vi "Flatten Cluster To CfgTable.vi"(8 "error in (no error)":errorcluster, 11 "Cluster Configuration Typedef":variant) -> (0 "error out":errorcluster, 3 "CfgTable Row":string[](array[string]))   [LabVIEW 2017, in "ClusterCfgTable.lvlib"]
uses:
  ClusterCfgTable.lvlib
panel:
  in  "ConfigStrings Typedef":string[](array[string])
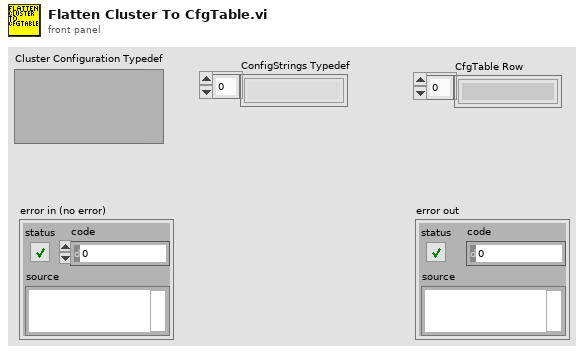
[diagram p1: front panel]
types:
  T1 = typedef "Type Descriptor Enumeration__ogtk.ctl" = enum8{"<Null>", "I8", "I16", "I32", "I64", "U8", "U16", "U32", "U64", "SGL", "DBL", "EXT", "CSG", "CDB", "CXT", "0x0F", "0x10", "0x11", "0x12", "0x13", "0x14", "Enum U8", "Enum U16", "Enum U32", "Enum U64", "SGL PQ", "DBL PQ", "EXT PQ", "CSG PQ", "CDB PQ", "CXT PQ", "0x1F", "0x20", "Boolean", "0x22", "0x23", "0x24", "0x25", "0x26", "0x27", "0x28", "0x29", "0x2A", "0x2B", "0x2C", "0x2D", "0x2E", "0x2F", "String", "0x31", "Path", "Pict", "0x34", "0x35", "0x36", "DAQ", "0x38", "0x39", "0x3A", "0x3B", "0x3C", "0x3D", "0x3E", "0x3F", "Array", "0x41", "0x42", "0x43", "0x44", "0x45", "0x46", "0x47", "0x48", "0x49", "0x4A", "0x4B", "0x4C", "0x4D", "0x4E", "0x4F", "Cluster", "0x51", "0x52", "Variant", "Waveform", "0x55", "0x56", "0x57", "0x58", "0x59", "0x5A", "0x5B", "0x5C", "0x5D", "0x5E", "0x5F", "0x60", "0x61", "0x62", "0x63", "0x64", "0x65", "0x66", "0x67", "0x68", "0x69", "0x6A", "0x6B", "0x6C", "0x6D", "0x6E", "0x6F", "Refnum"}
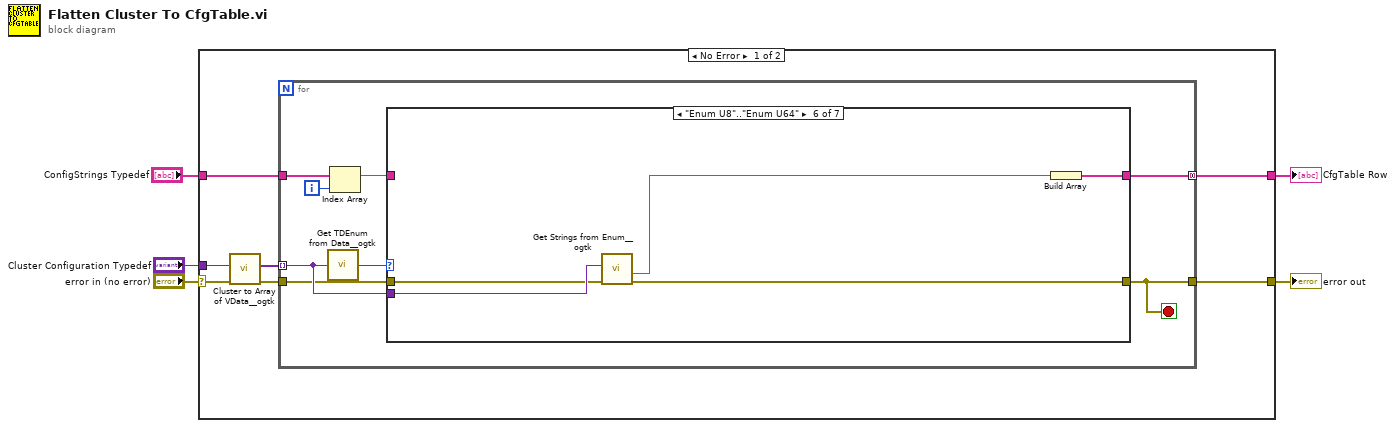
[diagram p0: block diagram]
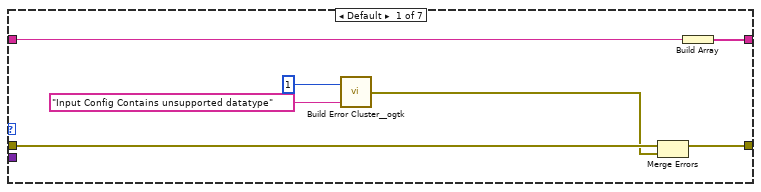
[diagram p2: hidden frame]
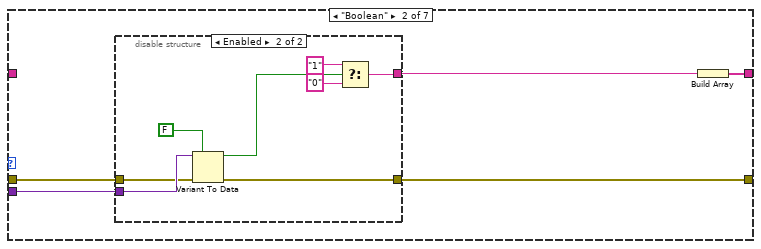
[diagram p3: hidden frame]
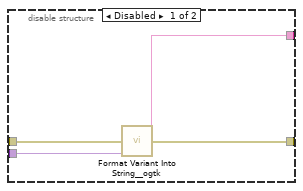
[diagram p4: hidden frame]
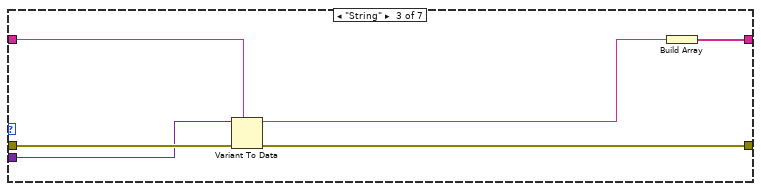
[diagram p5: hidden frame]
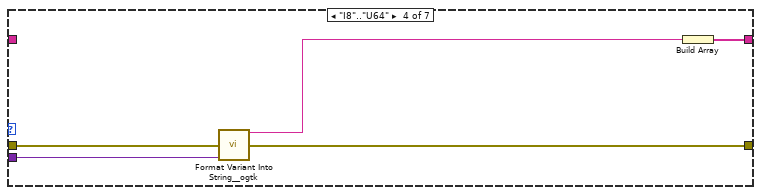
[diagram p6: hidden frame]
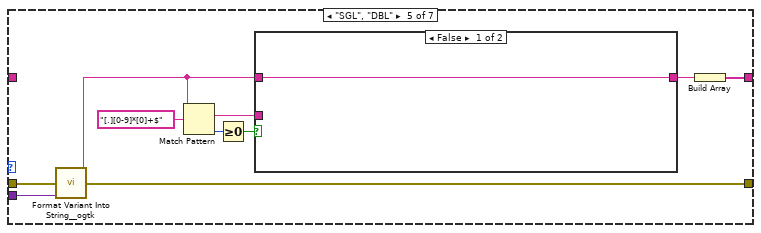
[diagram p7: hidden frame]
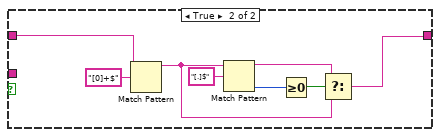
[diagram p8: hidden frame]
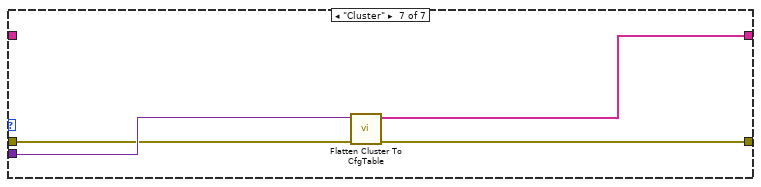
[diagram p9: hidden frame]
diagram:
  n1 = case shown="No Error" "error in (no error)" {
    selector: "error in (no error)" -> [w10 w85]
    tunnel: [w12 w85] -> w5
    tunnel: "Cluster Configuration Typedef" -> [w8 _]
    tunnel: [w7 w84] -> w2
    tunnel: "ConfigStrings Typedef" -> [w6 w84]
    frame No Error {
      n2 = call <userlib>:"Cluster to Array of VData__ogtk.vi"("error in (no error)"=w10, "Cluster"=w8) -> ("error out"=w11:errorcluster, "Array of VData"=w9:variant[])  [unwired: 8 in]
      n3 = for {
        tunnel: w9 -> [w19] mode=indexing
        tunnel: w11 -> [w18]
        tunnel: [w17] -> w12
        tunnel: [w16] -> w7 mode=concatenating
        tunnel: w6 -> [w15]
        i -> [w13]
        stop <- w17 stop-if-true
        n4 = call <userlib>:"Get TDEnum from Data__ogtk.vi"("Data"=w19) -> ("Type Descriptor Enumeration"=w20:T1)  [unwired: 4 in]
        n5 = Index Array(array=w15, index=w13) -> (element=w14:string)
        n6 = case shown="\"Enum U8\"..\"Enum U64\"" w20 {
          tunnel: w19 -> [_ w31 w48 w53 w59 w79 w83]
          tunnel: w18 -> [w27 w32 w50 w55 w60 w78 w81]
          tunnel: [w26 w29 w49 w54 w58 w76 w80] -> w17
          tunnel: [w21 w28 w45 w51 w56 w75 w82] -> w16
          tunnel: w14 -> [w22 _ w47 _ _ _ _]
          frame Default {
            n7 = call <userlib>:"Build Error Cluster__ogtk.vi"("String to Prepend to source (\"\")"="Input Config Contains unsupported datatype" ("String to Prepend to source (\"\")"), "code"=1) -> ("error out"=w25:errorcluster)
            n8 = Merge Errors(w27, w25) -> (w26:errorcluster)
            n9 = Build Array(w22) -> (w21:string[])
          }
          frame "Boolean" {
            n10 = disable-structure shown="Enabled" {
              disable-tunnel: w31 -> [w36 w44]
              disable-tunnel: w32 -> [w35 w43]
              disable-tunnel: [w34 w42] -> w29
              disable-tunnel: [w33 w39] -> w30
              frame Disabled {
                n11 = call <userlib>:"Format Variant Into String__ogtk.vi"("error in (no error)"=w35, "Variant"=w36) -> ("Output String"=w33:string, "error out"=w34:errorcluster)  [unwired: 12 in]
              }
              frame Enabled {
                n12 = Variant To Data(error in=w43, type=FALSE, Variant=w44) -> (data=w40:bool, error out=w42:errorcluster)
                n13 = Select(t="1", s=w40, f="0") -> (s? t:f=w39:string)
              }
            }
            n14 = Build Array(w30) -> (w28:string[])
          }
          frame "String" {
            n15 = Variant To Data(error in=w50, type=w47, Variant=w48) -> (data=w46:string, error out=w49:errorcluster)
            n16 = Build Array(w46) -> (w45:string[])
          }
          frame "I8".."U64" {
            n17 = call <userlib>:"Format Variant Into String__ogtk.vi"("error in (no error)"=w55, "Variant"=w53) -> ("Output String"=w52:string, "error out"=w54:errorcluster)  [unwired: 12 in]
            n18 = Build Array(w52) -> (w51:string[])
          }
          frame "SGL", "DBL" {
            n19 = call <userlib>:"Format Variant Into String__ogtk.vi"("error in (no error)"=w60, "Variant"=w59) -> ("Output String"=w62:string, "error out"=w58:errorcluster)  [unwired: 12 in]
            n20 = Match Pattern(string=w62, regular expression="[.][0-9]*[0]+$") -> (match substring=w61:string, offset past match=w64:i32)  [unwired: 1 in, 2 out]
            n21 = Greater Or Equal To 0?(x=w64) -> (x >= 0?=w63:bool)
            n22 = case shown="False" w63 {
              tunnel: [w66 w74] -> w57
              tunnel: w62 -> [w66 w72]
              tunnel: w61 -> [_ _]
              frame False {
              }
              frame True {
                n23 = Match Pattern(string=w72, regular expression="[0]+$") -> (before substring=w71:string)  [unwired: 1 in, 3 out]
                n24 = Match Pattern(string=w71, regular expression="[.]$") -> (before substring=w67:string, offset past match=w69:i32)  [unwired: 1 in, 2 out]
                n25 = Greater Or Equal To 0?(x=w69) -> (x >= 0?=w68:bool)
                n26 = Select(t=w67, s=w68, f=w71) -> (s? t:f=w74:string)
              }
            }
            n27 = Build Array(w57) -> (w56:string[])
          }
          frame "Enum U8".."Enum U64" {
            n28 = call <userlib>:"Get Strings from Enum__ogtk.vi"("error in (no error)"=w78, "Enum"=w79) -> ("error out"=w76:errorcluster, "String Value"=w77:string)  [unwired: 6 in, 2 out]
            n29 = Build Array(w77) -> (w75:string[])
          }
          frame "Cluster" {
            n30 = call "Flatten Cluster To CfgTable.vi"("error in (no error)"=w81, "Cluster Configuration Typedef"=w83) -> ("error out"=w80:errorcluster, "CfgTable Row"=w82:string[])  [unwired: 8 in]
          }
        }
      }
    }
    frame Error {
    }
  }
  "CfgTable Row" <- w2
  "error out" <- w5
